vi "FA_Delete.vi"(6 "Error In":errorcluster, 8 "Special Type":T1) -> (0 "Error Out":errorcluster)   [LabVIEW 2014, in "FA_LocalStore.lvlib"]
doc: "Removes the XML file reference from the array, deletes the Special Type's directory and all files contained within that directory. This VI does not do anything to the eTag INI file."
uses:
  FA_LocalStore.lvlib
  FA_LSSpecialTypes.ctl
  FA_LSCollections.ctl
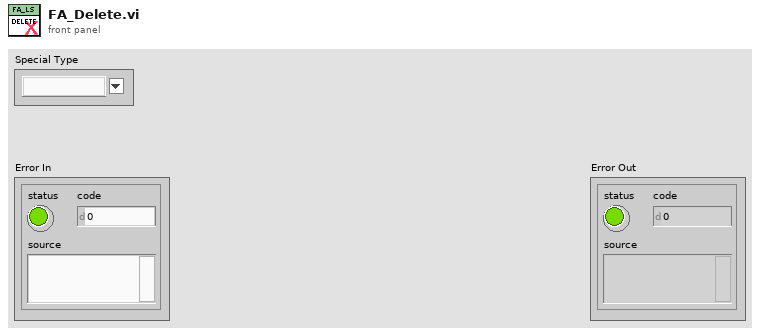
[diagram p1: front panel]
types:
  T1 = typedef "FA_LocalStore.lvlib/FA_LSSpecialTypes.ctl" = string
  T2 = typedef "FA_LocalStore.lvlib/FA_LSCollections.ctl" = enum16{"Config", "ConfigItem", "FA_eTag", "FA_PlugIn"}
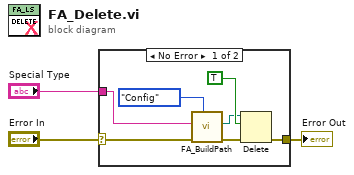
[diagram p0: block diagram]
diagram:
  n1 = case shown="No Error" "Error In" {
    selector: "Error In" -> [w5 w11]
    tunnel: [w10 w11] -> w1
    tunnel: "Special Type" -> [w9 _]
    frame No Error {
      n2 = call "FA_BuildPath.vi"("LSCollections"=FA_LSCollections."Config", "error in (no error)"=w5, "Special Type"=w9) -> ("error out"=w7:errorcluster, "directory path"=w4:path)  [unwired: 6 in, 1 out]
      n3 = Delete(path (use dialog)=w4, entire hierarchy (F)=TRUE, error in=w7) -> (error out=w10:errorcluster)  [unwired: 2 in, 2 out]
    }
    frame Error {
    }
  }
  "Error Out" <- w1
